vi "csv.vi"() -> ()   [LabVIEW 2017]
panel:
  out "size (in bytes)":i64
  out "offset (in bytes) 2":i64
  out "error out 2":errorcluster
  out "offset (in bytes)":i64
  in  "String":string
  out "error out":errorcluster
  out "path":path
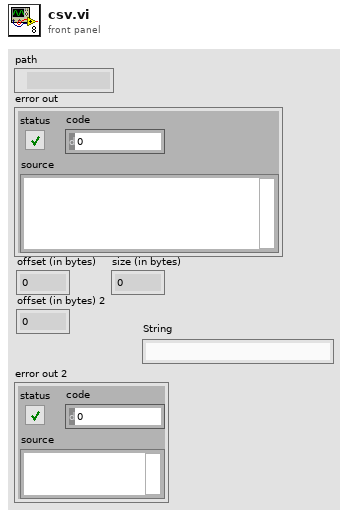
[diagram p1: front panel]
types:
  T1 = enum16{"open", "replace", "create", "open or create", "replace or create", "replace or create with confirmation"}
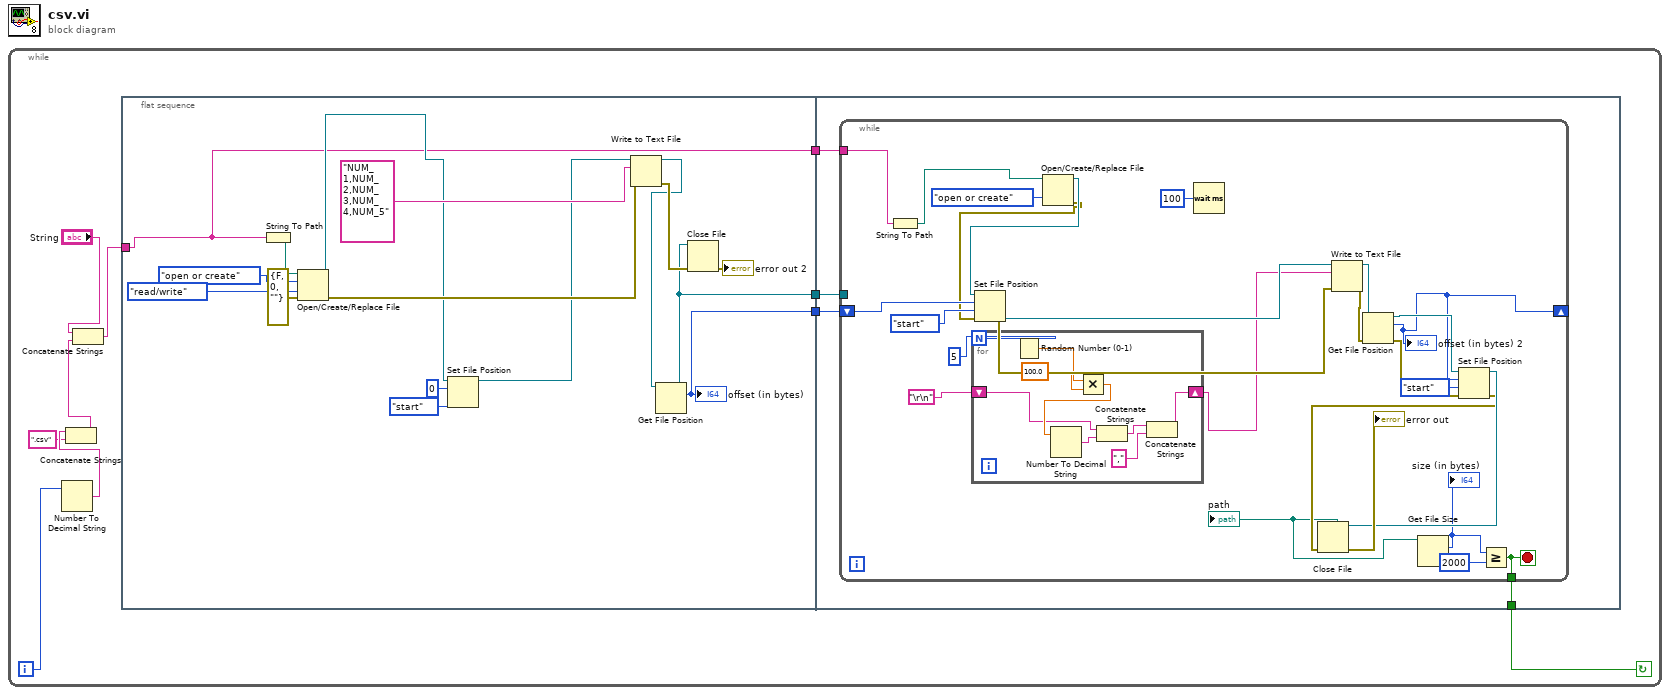
[diagram p0: block diagram]
diagram:
  n1 = while {
    i -> [w7]
    stop <- w8 continue-if-true
    n2 = Number To Decimal String(number=w7) -> (decimal integer string=w6:string)  [unwired: 1 in]
    n3 = Concatenate Strings(w6, ".csv" ("string")) -> (w4:string)
    n4 = Concatenate Strings("String", w4) -> (w2:string)
    n5 = flat-sequence {
      tunnel: [w15] -> w10
      tunnel: [w12] -> w9
      tunnel: w2 -> [w11]
      tunnel: [w11] -> w1
      tunnel: w10 -> [w30]
      tunnel: w9 -> [w29]
      tunnel: [w28] -> w8
      tunnel: w1 -> [w27]
      frame #0 {
        n6 = String To Path(string=w11) -> (path=w23:path)
        n7 = Open/Create/Replace File(file path (use dialog)=w23, error in=errorcluster {"status"=FALSE, "code"=0, "source"=""}, operation (0:open)=T1."open or create", access (0:read/write)=enum16{"read/write", "read-only", "write-only"}."read/write") -> (refnum out=w18:refnum<file>, error out=w20:errorcluster)  [unwired: 2 in, 1 out]
        n8 = Set File Position(offset (in bytes) (0)=i64 0, refnum=w18, from (0:start)=enum16{"start", "end", "current"}."start") -> (refnum out=w17:refnum<file>)  [unwired: 1 in, 1 out]
        n9 = Write to Text File(file (use dialog)=w17, text="NUM_1,NUM_2,NUM_3,NUM_4,NUM_5", error in=w20) -> (refnum out=w19:refnum<file>, error out=w22:errorcluster)  [unwired: 1 in, 1 out]
        n10 = Get File Position(7:w19) -> (2:w15:i64, 3:w12:refnum<file>)  [unwired: 1 in, 1 out]
        "offset (in bytes)" <- w15
        n11 = Close File(refnum=w12, error in=w22) -> (error out=→"error out 2":errorcluster)  [unwired: 1 out]
      }
      frame #1 {
        n12 = while {
          tunnel: w29 -> [_]
          shift-right: [w38] -> _
          shift-left: w30 -> [w52]
          tunnel: [w33] -> w28
          tunnel: w27 -> [w31]
          stop <- w33 stop-if-true
          n13 = String To Path(string=w31) -> (path=w32:path)
          n14 = for {
            N: 5 -> [_]
            shift-right: [w59] -> w39
            shift-left: "\r\n" -> [w60]
            n15 = Random Number (0-1)() -> (number: 0 to 1=w64:dbl)
            n16 = Multiply(x=w64, y=100.0) -> (x*y=w62:dbl)
            n17 = Number To Decimal String(number=w62) -> (decimal integer string=w61:string)  [unwired: 1 in]
            n18 = Concatenate Strings(w60, w61) -> (w58:string)
            n19 = Concatenate Strings(w58, "," ("string")) -> (w59:string)
          }
          n20 = Open/Create/Replace File(file path (use dialog)=w32, operation (0:open)=T1."open or create") -> (refnum out=w50:refnum<file>, error out=w48:errorcluster)  [unwired: 4 in, 1 out]
          n21 = Set File Position(offset (in bytes) (0)=w52, refnum=w50, from (0:start)=enum16{"start", "end", "current"}."start", error in=w48) -> (refnum out=w54:refnum<file>, error out=w53:errorcluster)
          n22 = Wait (ms)(milliseconds to wait=u32 100) -> ()  [unwired: 1 out]
          n23 = Write to Text File(file (use dialog)=w54, text=w39, error in=w53) -> (refnum out=w47:refnum<file>, error out=w46:errorcluster)  [unwired: 1 in, 1 out]
          n24 = Get File Position(4:w46, 7:w47) -> (0:w43:errorcluster, 2:w38:i64, 3:w45:refnum<file>)
          "offset (in bytes) 2" <- w38
          n25 = Set File Position(offset (in bytes) (0)=w38, refnum=w45, from (0:start)=enum16{"start", "end", "current"}."start", error in=w43) -> (refnum out=w44:refnum<file>, error out=w42:errorcluster)
          n26 = Close File(refnum=w44, error in=w42) -> (path=w37:path, error out=→"error out":errorcluster)
          "path" <- w37
          n27 = Get File Size(file=w37) -> (size (in bytes)=w36:i64)  [unwired: 1 in, 2 out]
          "size (in bytes)" <- w36
          n28 = Greater Or Equal?(x=w36, y=i64 2000) -> (x >= y?=w33:bool)
        }
      }
    }
  }
